vi "Setup(SubVI).vi"(8 "FM  Frequency":dbl, 9 "IQ Rate":dbl, 10 "ppm":i32, 11 "Device index":u32) -> (0 "error out":errorcluster, 2 "DevRefnum":u64, 3 "DevRefnum 2":u64)   [LabVIEW 2013]
uses:
  <instrlib>/rtlsdr/rtlsdr.lvlib
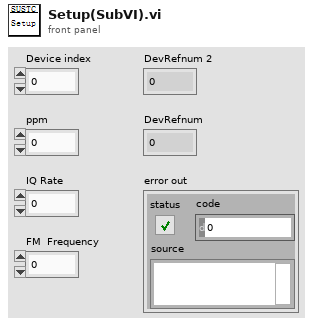
[diagram p1: front panel]
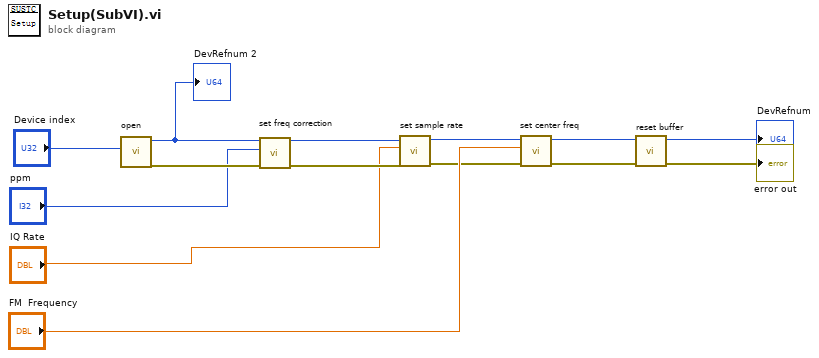
[diagram p0: block diagram]
diagram:
  n1 = call <instrlib>:"open.vi"("index"="Device index") -> ("error out"=w13:errorcluster, "DevRefnum"=w6:u64)  [unwired: 9 in]
  "DevRefnum 2" <- w6
  n2 = call <instrlib>:"set freq correction.vi"("error in (no error)"=w13, "ppm"="ppm") -> ("error out"=w12:errorcluster)  [unwired: 7 in, 2 out]
  n3 = call <instrlib>:"set sample rate.vi"("error in (no error)"=w12, "rate"="IQ Rate", "DevRefnum"=w6) -> ("error out"=w4:errorcluster, "DevRefnum"=w2:u64)  [unwired: 6 in, 1 out]
  n4 = call <instrlib>:"set center freq.vi"("error in (no error)"=w4, "freq"="FM  Frequency", "DevRefnum"=w2) -> ("error out"=w5:errorcluster, "DevRefnum"=w3:u64)  [unwired: 6 in, 1 out]
  n5 = call <instrlib>:"reset buffer.vi"("error in (no error)"=w5, "DevRefnum"=w3) -> ("error out"=→"error out":errorcluster, "DevRefnum"=→"DevRefnum":u64)  [unwired: 8 in]
